vi "close.vi"(8 "error in (no error)":errorcluster, 11 "Analog_Input (in)":refnum<class "Analog_Input.lvclass">) -> (0 "error out":errorcluster, 3 "Analog_Input":refnum<class "Analog_Input.lvclass">)   [LabVIEW 2013, in "Analog_Input.lvclass"]
uses:
  Analog_Input.lvclass
  Analog_Input.lvclass/Analog_Input.ctl
  Globals.vi
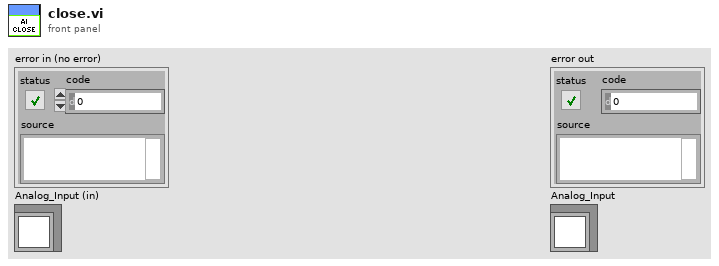
[diagram p1: front panel]
types:
  T1 = typedef "Experiment.lvclass/states.ctl" = enum16{"run", "pause", "shutdown gracefully", "halt immediately", "waiting for connection", "waiting for command"}
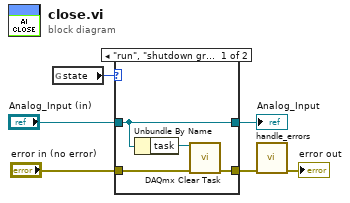
[diagram p0: block diagram]
diagram:
  n1 = global read "Globals.vi" "state"() -> (w4:T1)
  n2 = case shown="\"run\", \"shutdown gracefully\"" w4 {
    tunnel: "error in (no error)" -> [w8 w12]
    tunnel: [w10 w12] -> w6
    tunnel: "Analog_Input (in)" -> [w7 w11]
    tunnel: [w7 w11] -> w1
    frame "run", "shutdown gracefully" {
      n3 = Unbundle By Name(w7) -> ("task"=w9:refnum<k21>)
      n4 = call <vilib>:"DAQmx Clear Task.vi"("task in"=w9, "error in"=w8) -> ("error out"=w10:errorcluster)  [unwired: 13 in]
    }
    frame Default {
    }
  }
  "Analog_Input" <- w1
  n5 = call "handle_errors.vi"("error in (no error)"=w6) -> ("error out"=→"error out":errorcluster)  [unwired: 14 in]
